vi "CSVExample_S.vi"(0 "imageId":string, 1 "weight":string, 2 "rfid":string) -> ()   [LabVIEW 2019]
doc: "Takes in the RFID, Weight and Image name to stored in a location (currently it is stored in a csv file in the same folder as the grandparent VI)"
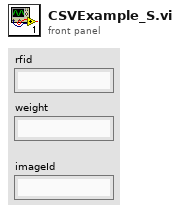
[diagram p1: front panel]
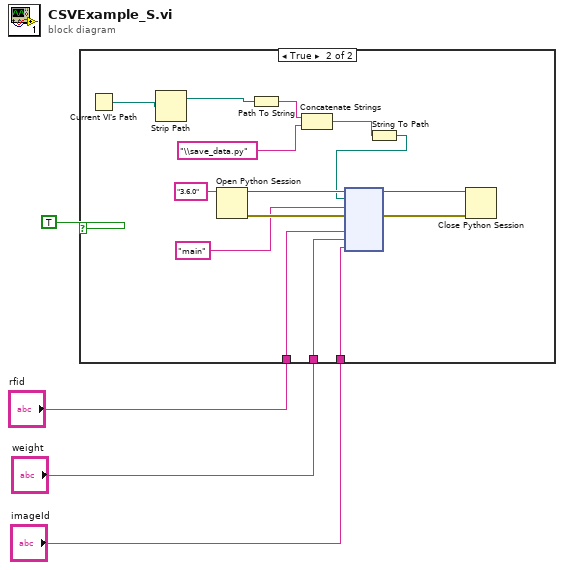
[diagram p0: block diagram]
diagram:
  n1 = case shown="True" TRUE {
    tunnel: "rfid" -> [_ w13]
    tunnel: "weight" -> [_ w12]
    tunnel: "imageId" -> [_ w11]
    frame False {
    }
    frame True {
      n2 = Current VI's Path() -> (path=w10:path)
      n3 = Strip Path(path=w10) -> (stripped path=w9:path)  [unwired: 1 out]
      n4 = Open Python Session(python version="3.6.0" ("Python version")) -> (session out=w19:refnum<k35>, error out=w18:errorcluster)  [unwired: 2 in]
      n5 = Path To String(path=w9) -> (string=w7:string)
      n6 = Concatenate Strings(w7, "\\save_data.py") -> (w6:string)
      n7 = String To Path(string=w6) -> (path=w5:path)
      n8 = node(w19, w5, "main" ("function name"), w18, w13, w12, w11) -> (w16:refnum<k35>, w17:errorcluster)  [unwired: 5 in, 2 out]
      n9 = Close Python Session(session in=w16, error in=w17) -> ()  [unwired: 1 out]
    }
  }
